vi "pdv_usb1.vi"() -> ()   [LabVIEW 2010]
uses:
  <vilib>/Utility/error.llb/DialogType.ctl
  70user.lib/TheSigTab.vi
  <vilib>/Utility/config.llb/Read Key (U32).vi
  <vilib>/Utility/config.llb/Read Key (String).vi
  <vilib>/addons/database/Connection.llb/DB Tools Open Connec (Path).vi
  <vilib>/addons/database/Connection.llb/Conn Get Properties.vi
  <vilib>/Utility/config.llb/Write Key (Double).vi
  <vilib>/Utility/config.llb/Write Key (U32).vi
  <vilib>/Utility/config.llb/Write Key (Boolean).vi
  <vilib>/Utility/config.llb/Write Key (String).vi
  <vilib>/addons/database/NI_Database_API.lvlib
  <vilib>/Utility/config.llb/NI_LVConfig.lvlib
panel:
  in  "OK Button":bool
  in  "Tab Control":enum32{"Таблица", "Графики"}(tab)
  in  "Table":string[][](table) caption="Результаты измерений"
  out "WChart":sgl[][](graph) caption="Q(R=0.5)"
  in  "ScopeToo":bool caption="Сохранять осциллограммы"
  in  "m_s":u16(ring) items=["мин", "сек"]
  in  "CurvesToo":bool caption="Сохранять графики"
  in  "AcqureTime":dbl caption="опроса" format="%#.3g"
  out "ExtDev":bool caption="Выносной модуль"
  in  "SaveTime":dbl=1.0 caption="мин" min=1.0 max=120.0
  out "Slide":u8(slide) scale=0.0..100.0
  in  "Continuosly":bool caption="Периодически"
  in  "SaveNow":bool caption="Однократно"
  in  "Loop":bool caption="Зациклить данные"
  out "Current time":timestamp caption="Время и Дата" format="%<%X\n%x>T"
  out "Tper":dbl caption="общая"
  in  "filter":bool caption="Фильтр\nперекрёстных помех"
  in  "Stop":bool
  # "Запись в базу данных"
  # "Продолжительность, с"
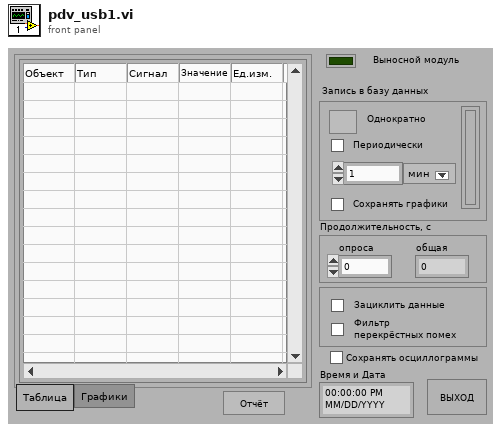
[diagram p1: front panel]
types:
  T1 = typedef "NI_LVConfig.lvlib/Config Data RefNum.ctl" = refnum<k1>
  T2 = typedef "NI_Database_API.lvlib/Conn ObjectReference.ctl" = refnum<k1>
  T3 = typedef "NI_Database_API.lvlib/Conn Properties.ctl" = cluster{"command timeout (s)":i32, "connection string":string, "default database":string, "provider":string}
  T4 = cluster{"Status":bool, "ViErrorNumber":u32, "ViName":string, "ViErrorString":string, "CinName":string, "CinErrorString":string}
  T5 = cluster{"VirtualSlot":u16, "ModuleName":string, "SerialNumber":string, "UsbSpeed":u8, "AvrVersion":string, "ModuleRevision":string, "DspType":string, "IsDacPresented":bool, "DspLoading":bool, "DspVersion":string, "DspClockout":u32, "AdcOffsetCoef":sgl[], "AdcScaleCoef":sgl[], "DacOffsetCoef":sgl[], "DacScaleCoef":sgl[]}
  T6 = cluster{"DllVersion":u32, "InterfaceType":u32, "InterfaceInstance":u32, "ModuleHandle":u32, "ReadBuffersParsArray":cluster{"Buffer":i16[], "ReadOv":u32, "ReadEvent":u32}[], "WriteBuffersParsArray":cluster{"Buffer":i16[], "WriteOv":u32, "WriteEvent":u32}[]}
  T7 = typedef "DialogType.ctl" = u16
  T8 = cluster{"Сигнал":string, "Тип":enum16{"Напряжение/Ток", "ЧР", "Температура", "Давление"}, "Object":string}[]
  T9 = cluster{"Сигнал":string, "Тип":enum16{"Напряжение/Ток", "ЧР", "Температура", "Давление"}, "Object":string}
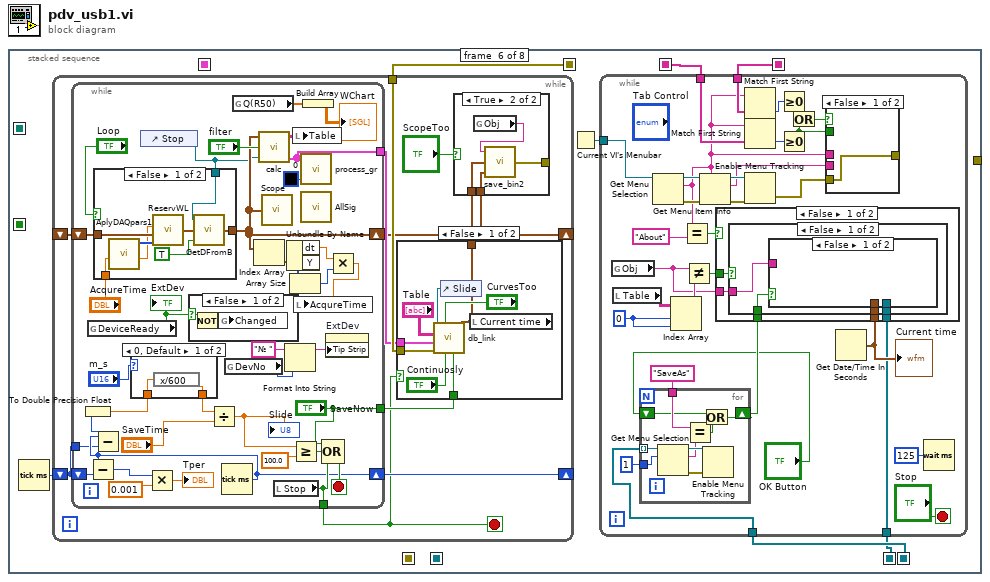
[diagram p0: block diagram]
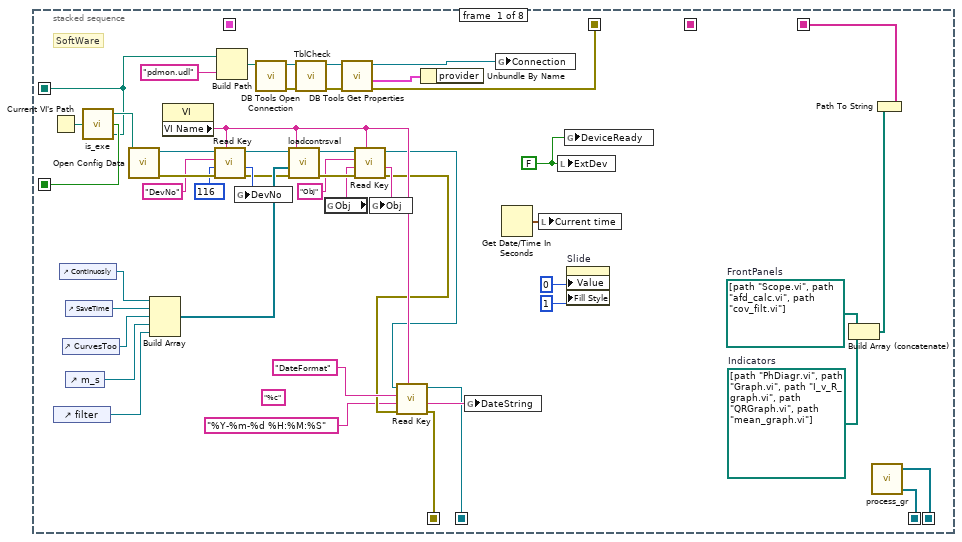
[diagram p2: hidden frame]
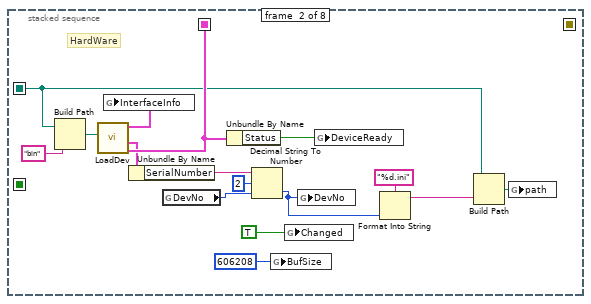
[diagram p3: hidden frame]
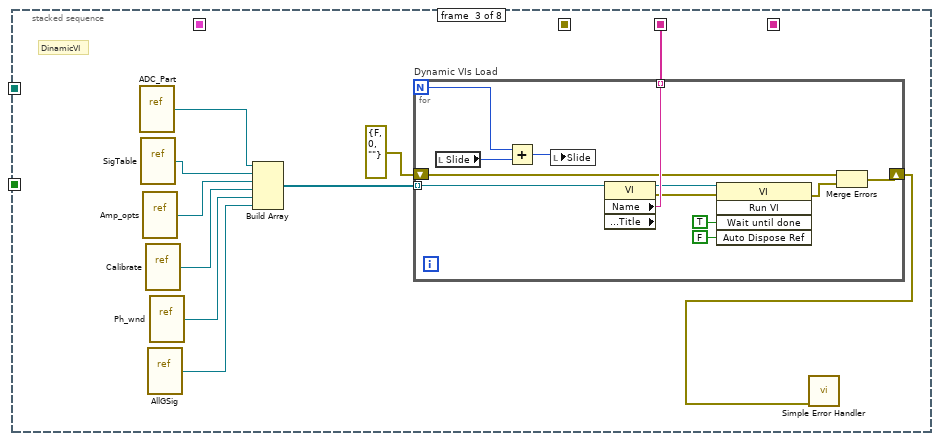
[diagram p4: hidden frame]
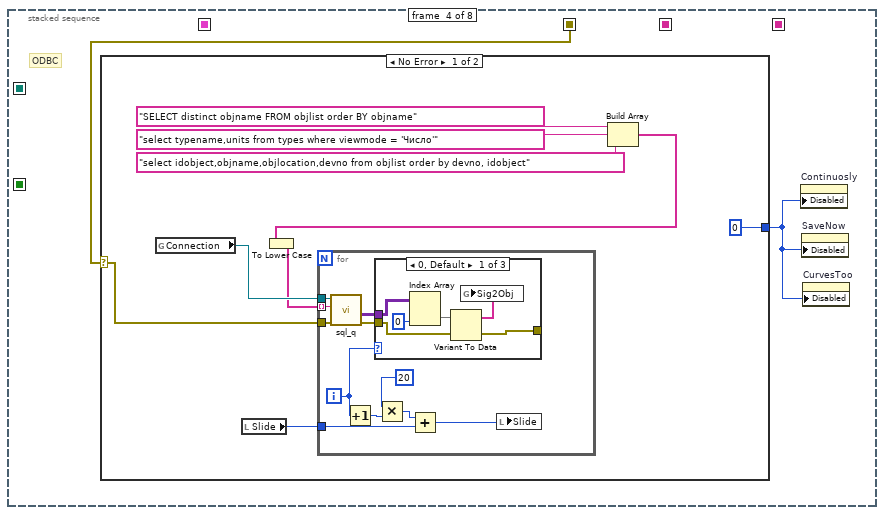
[diagram p5: hidden frame]
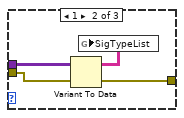
[diagram p6: hidden frame]
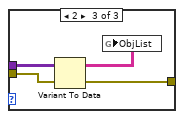
[diagram p7: hidden frame]
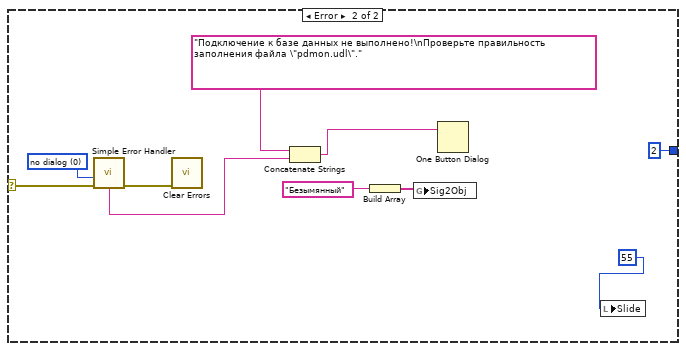
[diagram p8: hidden frame]
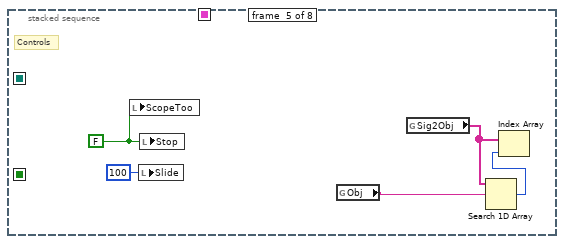
[diagram p9: hidden frame]
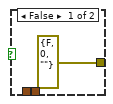
[diagram p10: hidden frame]
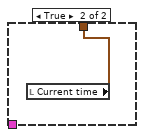
[diagram p11: hidden frame]
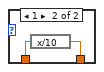
[diagram p12: hidden frame]
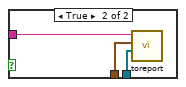
[diagram p15: hidden frame]
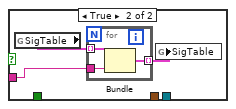
[diagram p16: hidden frame]
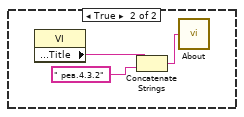
[diagram p17: hidden frame]
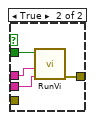
[diagram p18: hidden frame]
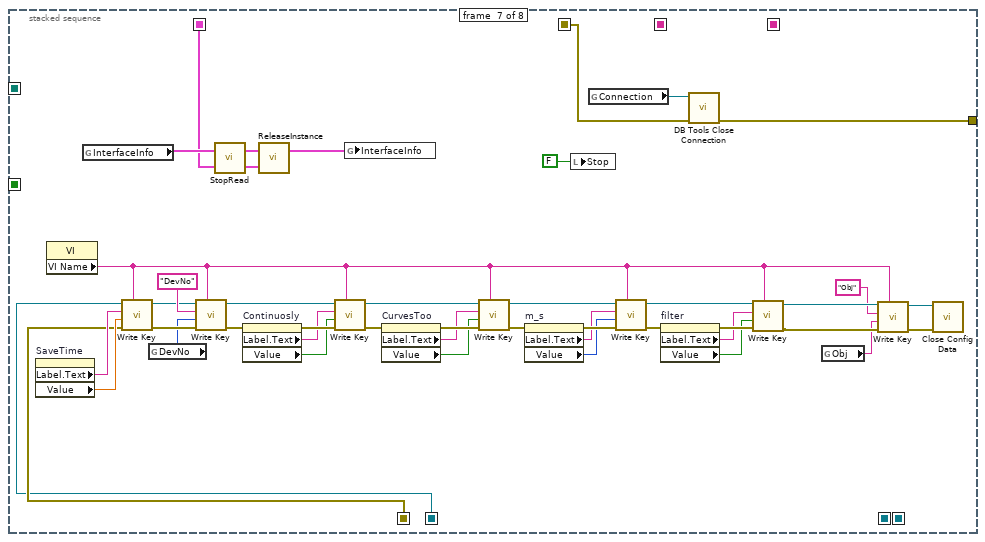
[diagram p19: hidden frame]
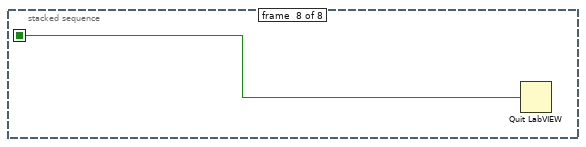
[diagram p20: hidden frame]
diagram:
  n1 = stacked-sequence {
    seq-local: [_ w61 _ _ _ _ _ _] -> [_ _ _ _ _ _ w324 _]
    seq-local: [w5 _ _ _ _ _ _ _] -> [_ _ _ w89 _ w144 w331 _]
    seq-local: [w41 _ _ _ _ _ _ _] -> [_ _ _ _ _ w142 _ _]
    seq-local: [_ _ w75 _ _ _ _ _] -> [_ _ _ _ _ w141 _ _]
    seq-local: [w46 _ _ _ _ _ _ _] -> [_ _ _ _ _ w139 _ _]
    seq-local: [w45 _ _ _ _ _ _ _] -> [_ _ _ _ _ w140 _ _]
    seq-local: [w16 _ _ _ _ _ _ _] -> [_ _ _ _ _ _ w316 _]
    seq-local: [w17 _ _ _ _ _ _ _] -> [_ _ _ _ _ _ w317 _]
    seq-local: [w28 _ _ _ _ _ _ _] -> [_ _ _ _ _ _ _ w332]
    seq-local: [w27 _ _ _ _ _ _ _] -> [_ w52 _ _ _ _ _ _]
    tunnel: [_ _ _ _ _ _ w328 _] -> _
    frame #0 {
      (unwired) "%c"
      w29 = FALSE ("ExtDev")
      w43 = path[] [path "PhDiagr.vi", path "Graph.vi", path "I_v_R_graph.vi", path "QRGraph.vi", path "mean_graph.vi"]  # Indicators
      w44 = path[] [path "Scope.vi", path "afd_calc.vi", path "cov_filt.vi"]  # FrontPanels
      # "SoftWare"
      n2 = Current VI's Path() -> (path=w49:path)
      n3 = control-ref of="filter"() -> (w22:refnum<vi>)
      n4 = control-ref of="Continuosly"() -> (w26:refnum<vi>)
      n5 = control-ref of="CurvesToo"() -> (w24:refnum<vi>)
      n6 = control-ref of="SaveTime"() -> (w25:refnum<vi>)
      n7 = control-ref of="m_s"() -> (w23:refnum<vi>)
      n8 = call "is_exe.vi"("path"=w49) -> ("actual path"=w27:path, "exe?"=w28:bool, "ini path"=w35:path)  [unwired: 2 in]
      n9 = call <vilib>:"Open Config Data.vi"("configuration file path"=w35) -> ("error out"=w33:errorcluster, "refnum"=w34:T1)  [unwired: 8 in, 1 out]
      n10 = Build Array(w26, w25, w24, w23, w22) -> (w21:refnum<vi>[])
      n11 = property class="VI"() -> ("VI Name"=w12:string)  [unwired: 2 in, 2 out]
      n12 = call-poly <vilib>:"Read Key.vi"("section"=w12, "error in (no error)"=w33, "default value"=u32 116 ("DevNo"), "key"="DevNo", "refnum"=w34) -> ("error out"=w20:errorcluster, "value"=w30:u32, "refnum out"=w15:T1)  [unwired: 3 in, 1 out]
      n13 = Build Path(base path=w27, name or relative path="pdmon.udl") -> (appended path=w47:path)
      n14 = global write "TheSigTab.vi" "DevNo"(w30) -> ()
      n15 = call-poly <vilib>:"DB Tools Open Connection.vi"("connection information"=w47) -> ("error out"=w39:errorcluster, "connection reference"=w40:T2)  [unwired: 7 in]
      n16 = call "loadcontrsval.vi"("error in"=w20, "Array"=w21, "Section"=w12, "refnum in"=w15) -> ("error out"=w13:errorcluster, "refnum out"=w14:T1)  [unwired: 2 in]
      n17 = call "TblCheck.vi"("error in"=w39, "connection reference"=w40) -> ("error out"=w6:errorcluster, "conn ref out"=w4:T2)  [unwired: 3 in, 1 out]
      n18 = global read "TheSigTab.vi" "Obj"() -> (w11:string)
      n19 = call-poly <vilib>:"DB Tools Get Properties.vi"("error in (no error)"=w6, "connection reference"=w4) -> ("error out"=w5:errorcluster, "connection properties"=w2:T3, "connection reference out"=w3:T2)  [unwired: 3 in]
      n20 = call-poly <vilib>:"Read Key.vi"("section"=w12, "error in (no error)"=w13, "default value"=w11, "key"="Obj", "refnum"=w14) -> ("error out"=w7:errorcluster, "value"=w10:string, "refnum out"=w8:T1)  [unwired: 3 in, 1 out]
      n21 = global write "TheSigTab.vi" "Obj"(w10) -> ()
      n22 = call-poly <vilib>:"Read Key.vi"("section"=w12, "error in (no error)"=w7, "default value"="%Y-%m-%d %H:%M:%S" ("time format string (%c)"), "key"="DateFormat", "refnum"=w8) -> ("error out"=w17:errorcluster, "value"=w18:string, "refnum out"=w16:T1)  [unwired: 3 in, 1 out]
      n23 = Unbundle By Name(w2) -> ()  [unwired: 1 out]
      n24 = global write "TheSigTab.vi" "DateString"(w18) -> ()
      n25 = global write "TheSigTab.vi" "Connection"(w3) -> ()
      n26 = Get Date/Time In Seconds() -> (seconds since 1Jan1904=w38:timestamp)
      n27 = local write "Current time"(w38) -> ()
      n28 = local write "ExtDev"(w29) -> ()
      n29 = global write "TheSigTab.vi" "DeviceReady"(w29) -> ()
      n30 = property on="Slide" class="Slide (strict)"("Value"=u8 0 ("Slide"), "Fill Style"=1) -> ()  [unwired: 2 in, 2 out]
      n31 = Build Array (concatenate)(w44, w43) -> (w42:path[])
      n32 = call "process_gr.vi"() -> ("WG refs"=w46:refnum<vi>[], "menu refs"=w45:refnum<k9>[])  [unwired: 4 in]
      n33 = Path To String(path=w42) -> (string=w41:string[])
    }
    frame #1 {
      # "HardWare"
      n34 = Build Path(base path=w52, name or relative path="bin") -> (appended path=w50:path)
      n35 = call "LoadDev.vi"("Path"=w50) -> ("ViStatus"=w61:T4, "ModuleInfo"=w60:T5, "InterfaceInfo"=w62:T6)  [unwired: 4 in]
      n36 = global write "TheSigTab.vi" "InterfaceInfo"(w62) -> ()
      n37 = Unbundle By Name(w60) -> ("SerialNumber"=w59:string)
      n38 = global read "TheSigTab.vi" "DevNo"() -> (w53:u32)
      n39 = Unbundle By Name(w61) -> ("Status"=w65:bool)
      n40 = Decimal String To Number(string=w59, offset=u32 2 ("initial scan location"), default (0L)=w53) -> (number=w54:u32)  [unwired: 1 out]
      n41 = global write "TheSigTab.vi" "BufSize"(u32 606208 ("BufSize")) -> ()
      n42 = global write "TheSigTab.vi" "Changed"(TRUE ("Changed")) -> ()
      n43 = global write "TheSigTab.vi" "DevNo"(w54) -> ()
      n44 = global write "TheSigTab.vi" "DeviceReady"(w65) -> ()
      n45 = Format Into String(format string="%d.ini", w54) -> (resulting string=w56:string)  [unwired: 2 in, 1 out]
      n46 = Build Path(base path=w52, name or relative path=w56) -> (appended path=w55:path)
      n47 = global write "TheSigTab.vi" "path"(w55) -> ()
    }
    frame #2 {
      # "DinamicVI"
      n48 = vi-ref "ADC_Part.vi"() -> (w74:refnum<vi>)
      n49 = vi-ref "SigTable.vi"() -> (w73:refnum<vi>)
      n50 = vi-ref "Amp_opts.vi"() -> (w72:refnum<vi>)
      n51 = vi-ref "Calibrate.vi"() -> (w71:refnum<vi>)
      n52 = vi-ref "AllGSig.vi"() -> (w69:refnum<vi>)
      n53 = vi-ref "Ph_wnd.vi"() -> (w70:refnum<vi>)
      n54 = Build Array(w74, w73, w72, w71, w70, w69) -> (w68:refnum<vi>[])
      n55 = for "Dynamic VIs Load" {
        N -> [w83]
        tunnel: [w86] -> w75 mode=indexing
        tunnel: w68 -> [w85] mode=indexing
        shift-right: [w78] -> w66
        shift-left: errorcluster {"status"=FALSE, "code"=0, "source"=""} ("error IO") -> [w76]
        n56 = local read "Slide"() -> (w84:u8)
        n57 = Add(x=w83, y=w84) -> (x+y=w87:i32)
        n58 = local write "Slide"(w87) -> ()
        n59 = property class="VI" props=["Name", "Front Panel.Title"](reference=w85) -> (reference out=w82:refnum<vi>, error out=w81:errorcluster, "Name"=w86:string)  [unwired: 1 in, 1 out]
        n60 = invoke class="VI" method="Run VI"(reference=w82, error in=w81, "Wait until done"=TRUE ("Wait Until Done"), "Auto Dispose Ref"=FALSE ("Auto Dispose Reference")) -> (error out=w77:errorcluster)  [unwired: 1 in, 4 out]
        n61 = Merge Errors(w76, w77) -> (w78:errorcluster)
      }
      n62 = call <vilib>:"Simple Error Handler.vi"("error in (no error)"=w66) -> ()  [unwired: 4 in, 5 out]
    }
    frame #3 {
      # "ODBC"
      n63 = case shown="No Error" w89 {
        selector: w89 -> [w94 w129]
        tunnel: [u8 0 ("Disabled") u8 2 ("Disabled")] -> w88
        frame No Error {
          n64 = global read "TheSigTab.vi" "Connection"() -> (w95:T2)
          n65 = local read "Slide"() -> (w93:u8)
          n66 = Build Array("SELECT distinct objname FROM objlist order BY objname", "select typename,units from types where viewmode = 'Число'", "select idobject,objname,objlocation,devno from objlist order by devno, idobject" ("table")) -> (w91:string[])
          n67 = To Lower Case(string=w91) -> (all lower case string=w90:string[])
          n68 = for {
            tunnel: w95 -> [w108]
            tunnel: w94 -> [w107]
            tunnel: w90 -> [w105] mode=indexing
            tunnel: w93 -> [w104]
            i -> [w101]
            n69 = call "sql_q.vi"("error in"=w107, "SQL query"=w105, "connect ref"=w108) -> ("error out"=w106:errorcluster, "recordset data"=w109:variant[][])  [unwired: 1 in, 2 out]
            n70 = Increment(x=w101) -> (x+1=w99:i32)
            n71 = case shown="0, Default" w101 {
              tunnel: w109 -> [w112 w119 w123]
              tunnel: w106 -> [w111 w117 w121]
              tunnel: [w110 w116 w120] -> _
              frame 0, Default {
                n72 = Index Array(array=w112, index (col)=0 ("disabled index (col)")) -> (element=w114:variant[])  [unwired: 1 in]
                n73 = Variant To Data(error in=w111, Variant=w114) -> (error out=w110:errorcluster, data=w113:string[])  [unwired: 1 in]
                n74 = global write "TheSigTab.vi" "Sig2Obj"(w113) -> ()
              }
              frame 1 {
                n75 = Variant To Data(error in=w117, Variant=w119) -> (error out=w116:errorcluster, data=w118:string[][])  [unwired: 1 in]
                n76 = global write "TheSigTab.vi" "SigTypeList"(w118) -> ()
              }
              frame 2 {
                n77 = Variant To Data(error in=w121, Variant=w123) -> (error out=w120:errorcluster, data=w122:string[][])  [unwired: 1 in]
                n78 = global write "TheSigTab.vi" "ObjList"(w122) -> ()
              }
            }
            n79 = Multiply(x=20, y=w99) -> (x*y=w102:i32)
            n80 = Add(x=w102, y=w104) -> (x+y=w103:i32)
            n81 = local write "Slide"(w103) -> ()
          }
        }
        frame Error {
          w128 = T7 0 items=["no dialog", "OK message", "continue or stop message", "OK message + warnings", "continue/stop + warnings"] ("type of dialog (OK msg:1)")
          n82 = call <vilib>:"Simple Error Handler.vi"("type of dialog (OK msg:1)"=w128, "error in (no error)"=w129) -> ("error out"=w127:errorcluster, "message"=w125:string)  [unwired: 3 in, 3 out]
          n83 = call <vilib>:"Clear Errors.vi"("error in (no error)"=w127) -> ()  [unwired: 6 in, 1 out]
          n84 = Concatenate Strings("Подключение к базе данных не выполнено!\nПроверьте правильность заполнения файла \"pdmon.udl\"." ("message"), w125) -> (w124:string)
          n85 = Build Array("Безымянный" ("table")) -> (w132:string[])
          n86 = global write "TheSigTab.vi" "Sig2Obj"(w132) -> ()
          n87 = One Button Dialog(message=w124) -> ()  [unwired: 1 in, 1 out]
          n88 = local write "Slide"(u8 55 ("Slide")) -> ()
        }
      }
      n89 = property on="Continuosly" class="Bool (strict)"("Disabled"=w88) -> ()  [unwired: 2 in, 2 out]
      n90 = property on="SaveNow" class="Bool"("Disabled"=w88) -> ()  [unwired: 2 in, 2 out]
      n91 = property on="CurvesToo" class="Bool (strict)"("Disabled"=w88) -> ()  [unwired: 2 in, 2 out]
    }
    frame #4 {
      w137 = FALSE ("Changed")
      # "Controls"
      n92 = local write "ScopeToo"(w137) -> ()
      n93 = local write "Slide"(u8 100 ("Slide")) -> ()
      n94 = local write "Stop"(w137) -> ()
      n95 = global read "TheSigTab.vi" "Obj"() -> (w134:string)
      n96 = global read "TheSigTab.vi" "Sig2Obj"() -> (w136:string[])
      n97 = Search 1D Array(1D array=w136, element=w134) -> (index of element=w135:i32)  [unwired: 1 in]
      n98 = Index Array(array=w136, index=w135) -> ()  [unwired: 1 out]
    }
    frame #5 {
      n99 = Tick Count (ms)() -> (millisecond timer value=w145:u32)
      n100 = while {
        shift-right: [w155] -> _
        shift-left: w145 -> [w152]
        shift-right: [w148] -> _
        shift-left: _ -> [w154]
        tunnel: w144 -> [w153]
        stop <- w149 stop-if-true
        n101 = while {
          shift-right: [w184] -> w148
          shift-left: w154 -> [w203]
          shift-right: [w198] -> w155
          shift-left: w152 -> [w204]
          tunnel: [w200] -> w149
          tunnel: w152 -> [w197]
          tunnel: ["SaveNow"] -> w151
          tunnel: [w190] -> w150
          stop <- w199 stop-if-true
          n102 = global read "TheSigTab.vi" "DeviceReady"() -> (w195:bool)
          "ExtDev" <- w195
          n103 = control-ref of="Stop"() -> (w178:refnum<vi>)
          n104 = case shown="False" "Loop" {
            tunnel: w203 -> [w220 w221]
            tunnel: [w217 w221] -> w184
            tunnel: "AcqureTime" -> [w214 _]
            tunnel: w178 -> [w213 _]
            frame False {
              n105 = call "AplyDAQpars1.vi"("AcqTimeIn"=w214) -> ("t1-t0"=w215:dbl, "Idxs"=w219:i32[])  [unwired: 5 in]
              n106 = call "ReservWL.vi"("Tags"=w219, "ArrayIn"=w220, "t1-t0"=w215) -> ("Array"=w218:waveform(i16)[])  [unwired: 1 in]
              n107 = call "GetDFromB.vi"("Control"=TRUE, "ArrayIn"=w218, "Bool Refnum"=w213) -> ("ArrayOut"=w217:waveform(i16)[])
            }
            frame True {
            }
          }
          n108 = case shown="False" w195 {
            selector: w195 -> [w212 _]
            frame False {
              n109 = Not(x=w212) -> (.not. x?=w211:bool)
              n110 = global write "TheSigTab.vi" "Changed"(w211) -> ()
            }
            frame True {
            }
          }
          n111 = Tick Count (ms)() -> (millisecond timer value=w198:u32)
          n112 = Subtract(x=w198, y=w204) -> (x-y=w194:u32)
          n113 = Subtract(x=w198, y=w197) -> (x-y=w196:u32)
          n114 = To Double Precision Float(number=w196) -> (double precision float=w173:dbl)
          n115 = case shown="0, Default" "m_s" {
            tunnel: w173 -> [w208 w210]
            tunnel: [w207 w209] -> w172
            frame 0, Default {
              n116 = expression code="x/600"(w208) -> (w207:dbl)
            }
            frame 1 {
              n117 = expression code="x/10"(w210) -> (w209:dbl)
            }
          }
          n118 = Multiply(x=w194, y=0.001 ("x")) -> (x*y=→"Tper":dbl)
          n119 = Divide(x=w172, y="SaveTime") -> (x/y=w188:dbl)
          "Slide" <- w188
          n120 = global read "TheSigTab.vi" "DevNo"() -> (w175:u32)
          n121 = global read "TheSigTab.vi" "Q(R50)"() -> (w170:sgl[])
          n122 = Index Array(array=w184) -> (element=w183:waveform(i16))  [unwired: 1 in]
          n123 = call "calc.vi"("Acquire"=w178, "filter"="filter", "ArrayIn"=w184) -> ("AllMeasures"=w190:cluster{"x0":dbl, "dx":dbl, "y":sgl[][]}[], "Values"=w206:string[][])  [unwired: 1 in]
          n124 = call "Scope.vi"("Array"=w184) -> ()
          n125 = local read "Stop"() -> (w200:bool)
          n126 = Format Into String(initial string="№ ", w175) -> (resulting string=w177:string)  [unwired: 2 in, 1 out]
          n127 = Unbundle By Name(w183) -> ("dt"=w181:dbl, "Y"=w182:i16[])
          n128 = Array Size(array=w182) -> (size(s)=w180:i32)
          n129 = Greater Or Equal?(x=w188, y=100.0 ("x")) -> (x >= y?=w185:bool)
          n130 = local write "Table"(w206) -> ()
          n131 = call "process_gr.vi"("Color Box"=u32 0, "AllMeasures"=w190) -> ()  [unwired: 2 in, 2 out]
          n132 = call "AllSig.vi"() -> ()  [unwired: 1 in]
          n133 = Build Array(w170) -> (→"WChart":sgl[][])
          n134 = Compound Arithmetic op=OR("SaveNow", w185, w200) -> (w199:bool)
          n135 = property on="ExtDev" class="Bool (strict)"("Tip Strip"=w177) -> ()  [unwired: 2 in, 2 out]
          n136 = Multiply(x=w181, y=w180) -> (x*y=w179:dbl)
          n137 = local write "AcqureTime"(w179) -> ()
        }
        n138 = case shown="False" w149 {
          tunnel: w153 -> [w168 _]
          tunnel: w151 -> [w167 _]
          tunnel: w150 -> [w165 _]
          tunnel: [w161 w169] -> w147
          frame False {
            n139 = control-ref of="Slide"() -> (w164:refnum<vi>)
            n140 = local read "Current time"() -> (w161:timestamp)
            n141 = call "db_link.vi"("Current time"=w161, "SaveNow"=w167, "Continuosly"="Continuosly", "SaveCurves?"="CurvesToo", "error in"=w168, "AllMeasures"=w165, "Table"="Table", "reference"=w164) -> ()  [unwired: 3 in, 1 out]
          }
          frame True {
            n142 = local read "Current time"() -> (w169:timestamp)
          }
        }
        n143 = case shown="True" "ScopeToo" {
          tunnel: [errorcluster {"status"=FALSE, "code"=0, "source"=""} ("error out") w160] -> _
          tunnel: w148 -> [_ w159]
          tunnel: w147 -> [_ w158]
          frame False {
          }
          frame True {
            n144 = global read "TheSigTab.vi" "Obj"() -> (w157:string)
            n145 = call "save_bin2.vi"("ArrayOut"=w159, "Current time"=w158, "Object"=w157) -> ("error out"=w160:errorcluster)
          }
        }
      }
      n146 = Current VI's Menubar() -> (w143:refnum<k9>)
      n147 = while {
        tunnel: w143 -> [w250]
        tunnel: w142 -> [w246]
        tunnel: w141 -> [w243]
        tunnel: w140 -> [w230]
        tunnel: w139 -> [w227]
        stop <- "Stop" stop-if-true
        w225 = 0 ("index (row)")
        n148 = global read "TheSigTab.vi" "Obj"() -> (w223:string)
        n149 = local read "Table"() -> (w226:string[][])
        n150 = for {
          tunnel: "SaveAs" -> [w258]
          tunnel: w230 -> [w257] mode=indexing
          tunnel: 1 ("ms timeout (200)") -> [w256]
          shift-right: [w254] -> w229
          shift-left: "OK Button" -> [w253]
          n151 = Get Menu Selection(0:w257, 1:w256) -> (5:w261:refnum<k9>, 6:w259:string, 8:w260:errorcluster)  [unwired: 2 in, 2 out]
          n152 = Equal?(x=w258, y=w259) -> (x = y?=w255:bool)
          n153 = Or(x=w253, y=w255) -> (x .or. y?=w254:bool)
          n154 = Enable Menu Tracking(2:w260, 4:w261) -> ()  [unwired: 1 in, 2 out]
        }
        n155 = Get Menu Selection(0:w250) -> (5:w249:refnum<k9>, 6:w236:string, 8:w242:errorcluster)  [unwired: 3 in, 2 out]
        n156 = Index Array(array=w226, index (row)=w225, index (col)=w225) -> (element=w224:string)
        n157 = Equal?(x=w236, y="About") -> (x = y?=w235:bool)
        n158 = Not Equal?(x=w223, y=w224) -> (x != y?=w233:bool)
        n159 = Get Menu Item Info(7:w236, 8:w242, 11:w249) -> (0:w241:errorcluster, 2:w245:string, 3:w248:refnum<k9>)  [unwired: 4 out]
        n160 = Match First String(2:w246, 3:w236) -> (0:w247:i32)  [unwired: 1 out]
        n161 = Match First String(2:w243, 3:w236) -> (0:w244:i32)  [unwired: 1 out]
        n162 = Enable Menu Tracking(2:w241, 4:w248) -> (0:w237:errorcluster)  [unwired: 1 in, 1 out]
        n163 = Greater Or Equal To 0?(x=w247) -> (x >= 0?=w240:bool)
        n164 = Greater Or Equal To 0?(x=w244) -> (x >= 0?=w239:bool)
        n165 = Or(x=w240, y=w239) -> (x .or. y?=w238:bool)
        n166 = case shown="False" w238 {
          tunnel: w245 -> [_ w287]
          tunnel: w236 -> [_ w286]
          tunnel: w239 -> [_ w285]
          tunnel: w237 -> [w283 _]
          tunnel: [w283 w284] -> _
          frame False {
          }
          frame True {
            n167 = call "RunVi.vi"("Title"=w287, "Name"=w286, "Run/JustOpen"=w285) -> ("error out"=w284:errorcluster)  [unwired: 4 in]
          }
        }
        n168 = Get Date/Time In Seconds() -> (seconds since 1Jan1904=w228:timestamp)
        "Current time" <- w228
        n169 = case shown="False" w235 {
          tunnel: w233 -> [w266 _]
          tunnel: w223 -> [w265 _]
          tunnel: w229 -> [w264 _]
          tunnel: w228 -> [w263 _]
          tunnel: w227 -> [w262 _]
          frame False {
            n170 = case shown="False" w266 {
              tunnel: w265 -> [w269 w274]
              tunnel: w264 -> [w270 _]
              tunnel: w263 -> [w268 _]
              tunnel: w262 -> [w267 _]
              frame False {
                n171 = case shown="False" w270 {
                  tunnel: w269 -> [_ w273]
                  tunnel: w268 -> [_ w272]
                  tunnel: w267 -> [_ w271]
                  frame False {
                  }
                  frame True {
                    n172 = call "toreport.vi"("WG"=w271, "Time Stamp"=w272, "Object"=w273) -> ()  [unwired: 5 in]
                  }
                }
              }
              frame True {
                n173 = global read "TheSigTab.vi" "SigTable"() -> (w276:T8)
                n174 = for {
                  tunnel: w276 -> [w279] mode=indexing
                  tunnel: w274 -> [w278]
                  tunnel: [w277] -> w275 mode=indexing
                  n175 = Bundle(cluster=w279, "Object"=w278) -> (w277:T9)  [unwired: 2 in]
                }
                n176 = global write "TheSigTab.vi" "SigTable"(w275) -> ()
              }
            }
          }
          frame True {
            n177 = property class="VI"() -> ("Front Panel Window:Title"=w282:string)  [unwired: 2 in, 2 out]
            n178 = Concatenate Strings(w282, " рев.4.3.2" ("input 1")) -> (w280:string)
            n179 = call "About.vi"("Revision Number"=w280) -> ()
          }
        }
        n180 = Wait (ms)(milliseconds to wait=u32 125) -> ()  [unwired: 1 out]
      }
    }
    frame #6 {
      n181 = property on="SaveTime" class="DigNum (strict)"() -> ("Label.Text"=w319:string, "Value"=w318:dbl)  [unwired: 2 in, 2 out]
      n182 = property class="VI"() -> ("VI Name"=w293:string)  [unwired: 2 in, 2 out]
      n183 = global read "TheSigTab.vi" "InterfaceInfo"() -> (w326:T6)
      n184 = call-poly <vilib>:"Write Key.vi"("section"=w293, "error in (no error)"=w317, "value"=w318, "key"=w319, "refnum"=w316) -> ("error out"=w320:errorcluster, "refnum out"=w321:T1)  [unwired: 4 in, 1 out]
      n185 = global read "TheSigTab.vi" "DevNo"() -> (w291:u32)
      n186 = call-poly <vilib>:"Write Key.vi"("section"=w293, "error in (no error)"=w320, "value"=w291, "key"="DevNo", "refnum"=w321) -> ("error out"=w315:errorcluster, "refnum out"=w313:T1)  [unwired: 4 in, 1 out]
      n187 = call "StopRead.vi"("ViStatusIn"=w324, "InterfaceInfoIn"=w326) -> ("ViStatusOut"=w323:T4, "InterfaceInfoOut"=w325:T6)
      n188 = property on="Continuosly" class="Bool (strict)"(error in=w315) -> (error out=w314:errorcluster, "Label.Text"=w312:string, "Value"=w311:bool)  [unwired: 1 in, 1 out]
      n189 = call "ReleaseInstance.vi"("ViStatusIn"=w323, "InterfaceInfoIn"=w325) -> ("InterfaceInfoOut"=w327:T6)  [unwired: 1 out]
      n190 = call-poly <vilib>:"Write Key.vi"("section"=w293, "error in (no error)"=w314, "value"=w311, "key"=w312, "refnum"=w313) -> ("error out"=w310:errorcluster, "refnum out"=w306:T1)  [unwired: 4 in, 1 out]
      n191 = global write "TheSigTab.vi" "InterfaceInfo"(w327) -> ()
      n192 = property on="CurvesToo" class="Bool (strict)"(error in=w310) -> (error out=w309:errorcluster, "Label.Text"=w308:string, "Value"=w307:bool)  [unwired: 1 in, 1 out]
      n193 = call-poly <vilib>:"Write Key.vi"("section"=w293, "error in (no error)"=w309, "value"=w307, "key"=w308, "refnum"=w306) -> ("error out"=w305:errorcluster, "refnum out"=w301:T1)  [unwired: 4 in, 1 out]
      n194 = property on="m_s" class="Ring (strict)"(error in=w305) -> (error out=w304:errorcluster, "Label.Text"=w297:string, "Value"=w292:u16)  [unwired: 1 in, 1 out]
      n195 = local write "Stop"(FALSE ("Stop")) -> ()
      n196 = global read "TheSigTab.vi" "Connection"() -> (w330:T2)
      n197 = call-poly <vilib>:"Write Key.vi"("section"=w293, "error in (no error)"=w304, "value"=w292, "key"=w297, "refnum"=w301) -> ("error out"=w303:errorcluster, "refnum out"=w300:T1)  [unwired: 4 in, 1 out]
      n198 = property on="filter" class="Bool (strict)"(error in=w303) -> (error out=w302:errorcluster, "Label.Text"=w299:string, "Value"=w298:bool)  [unwired: 1 in, 1 out]
      n199 = call <vilib>:"DB Tools Close Connection.vi"("error in (no error)"=w331, "connection reference"=w330) -> ("error out"=w328:errorcluster)  [unwired: 5 in]
      n200 = call-poly <vilib>:"Write Key.vi"("section"=w293, "error in (no error)"=w302, "value"=w298, "key"=w299, "refnum"=w300) -> ("error out"=w290:errorcluster, "refnum out"=w296:T1)  [unwired: 4 in, 1 out]
      n201 = global read "TheSigTab.vi" "Obj"() -> (w289:string)
      n202 = call-poly <vilib>:"Write Key.vi"("section"=w293, "error in (no error)"=w290, "value"=w289, "key"="Obj", "refnum"=w296) -> ("error out"=w294:errorcluster, "refnum out"=w295:T1)  [unwired: 4 in, 1 out]
      n203 = call <vilib>:"Close Config Data.vi"("error in (no error)"=w294, "refnum"=w295) -> ()  [unwired: 8 in, 2 out]
    }
    frame #7 {
      n204 = Quit LabVIEW(quit? (T)=w332) -> ()
    }
  }
